vi "MaxMin_4ch_v00.vi"(8 "Reset MaxMin?":T2, 9 "Min (-1)":T3, 10 "Max (-1)":T4, 11 "Error Signals":T1) -> (0 "Max":T4, 3 "Min":T3)   [LabVIEW 2013]
uses:
  Strict Type Defs/1BS3HD Max.ctl
  Strict Type Defs/1BS3HD Min.ctl
  Strict Type Defs/1BS3HD Reset MaxMin.ctl
  Strict Type Defs/1BS3HD Error Signals.ctl
panel:
  in  "Min 2":T3
  in  "Max typedef":T4
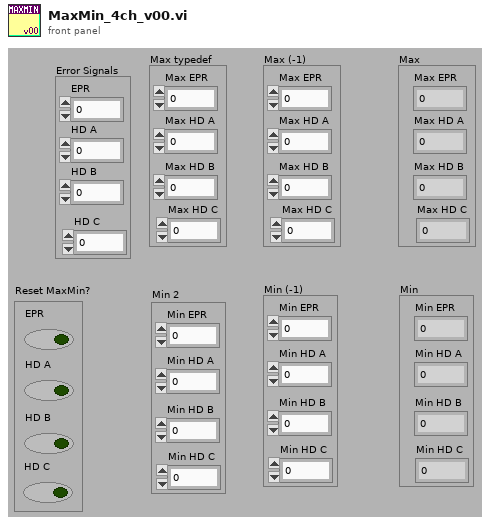
[diagram p1: front panel]
types:
  T1 = typedef "1BS3HD Error Signals.ctl" = cluster{"EPR":i16, "HD A":i16, "HD B":i16, "HD C":i16}
  T2 = typedef "1BS3HD Reset MaxMin.ctl" = cluster{"EPR":bool, "HD A":bool, "HD B":bool, "HD C":bool}
  T3 = typedef "1BS3HD Min.ctl" = cluster{"Min EPR":i16, "Min HD A":i16, "Min HD B":i16, "Min HD C":i16}
  T4 = typedef "1BS3HD Max.ctl" = cluster{"Max EPR":i16, "Max HD A":i16, "Max HD B":i16, "Max HD C":i16}
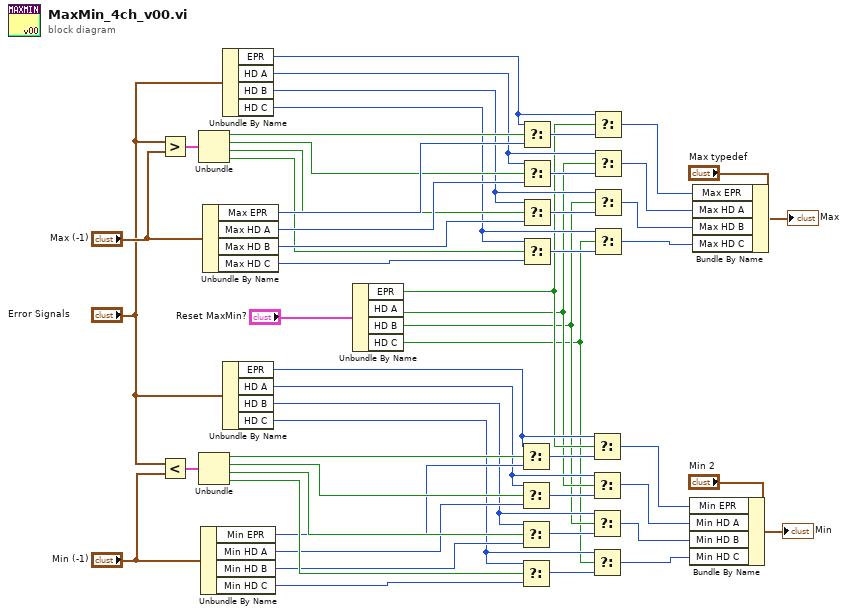
[diagram p0: block diagram]
diagram:
  n1 = Greater?(x="Error Signals", y="Max (-1)") -> (0:w45:cluster{bool, bool, bool, bool})
  n2 = Less?(x="Error Signals", y="Min (-1)") -> (x < y?=w31:cluster{bool, bool, bool, bool})
  n3 = Unbundle(w45) -> (w44:bool, w43:bool, w42:bool, w41:bool)
  n4 = Unbundle(w31) -> (w37:bool, w38:bool, w39:bool, w40:bool)
  n5 = Unbundle By Name("Min (-1)") -> ("Min EPR"=w33:i16, "Min HD A"=w34:i16, "Min HD B"=w35:i16, "Min HD C"=w36:i16)
  n6 = Unbundle By Name("Max (-1)") -> ("Max EPR"=w54:i16, "Max HD A"=w53:i16, "Max HD B"=w52:i16, "Max HD C"=w51:i16)
  n7 = Unbundle By Name("Error Signals") -> ("EPR"=w26:i16, "HD A"=w25:i16, "HD B"=w24:i16, "HD C"=w23:i16)
  n8 = Unbundle By Name("Error Signals") -> ("EPR"=w17:i16, "HD A"=w16:i16, "HD B"=w15:i16, "HD C"=w14:i16)
  n9 = Unbundle By Name("Reset MaxMin?") -> ("EPR"=w13:bool, "HD A"=w12:bool, "HD B"=w11:bool, "HD C"=w10:bool)
  n10 = Select(t=w17, s=w37, f=w33) -> (s? t:f=w21:i16)
  n11 = Select(t=w16, s=w38, f=w34) -> (s? t:f=w19:i16)
  n12 = Select(t=w15, s=w39, f=w35) -> (s? t:f=w20:i16)
  n13 = Select(t=w14, s=w40, f=w36) -> (s? t:f=w18:i16)
  n14 = Select(t=w26, s=w44, f=w54) -> (s? t:f=w27:i16)
  n15 = Select(t=w25, s=w43, f=w53) -> (s? t:f=w28:i16)
  n16 = Select(t=w24, s=w42, f=w52) -> (s? t:f=w29:i16)
  n17 = Select(t=w23, s=w41, f=w51) -> (s? t:f=w30:i16)
  n18 = Select(t=w17, s=w13, f=w21) -> (s? t:f=w2:i16)
  n19 = Select(t=w16, s=w12, f=w19) -> (s? t:f=w3:i16)
  n20 = Select(t=w15, s=w11, f=w20) -> (s? t:f=w4:i16)
  n21 = Select(t=w14, s=w10, f=w18) -> (s? t:f=w5:i16)
  n22 = Select(t=w26, s=w13, f=w27) -> (s? t:f=w6:i16)
  n23 = Select(t=w25, s=w12, f=w28) -> (s? t:f=w7:i16)
  n24 = Select(t=w24, s=w11, f=w29) -> (s? t:f=w8:i16)
  n25 = Select(t=w23, s=w10, f=w30) -> (s? t:f=w9:i16)
  n26 = Bundle By Name(cluster="Min 2", "Min EPR"=w2, "Min HD A"=w3, "Min HD B"=w4, "Min HD C"=w5) -> (→"Min":T3)
  n27 = Bundle By Name(cluster="Max typedef", "Max EPR"=w6, "Max HD A"=w7, "Max HD B"=w8, "Max HD C"=w9) -> (→"Max":T4)
